vi "Get points_pretrigger_box.vi"(7 "level":dbl=3.0 format="%#_13g", 8 "error in (no error)":errorcluster, 9 "Sample Rate":dbl=1000000.0 format="%.3p", 10 "Voltage Read":tag="Dev1/ai1") -> (0 "error out":errorcluster, 3 "data":dbl[](array[numeric]) format="%0.2f")   [LabVIEW 2017]
uses:
  <vilib>/DAQmx/read.llb/DAQmx Read (Analog 1D DBL 1Chan NSamp).vi
  <vilib>/DAQmx/create/channels.llb/DAQmx Create Channel (AI-Voltage-Basic).vi
  <vilib>/DAQmx/configure/timing.llb/DAQmx Timing (Sample Clock).vi
  <vilib>/DAQmx/configure/trigger.llb/DAQmx Reference Trigger (Analog Edge).vi
  <vilib>/DAQmx/miscellaneous.llb/DAQmx Fill In Error Info.vi
panel:
  out "Waveform Graph":dbl[](graph)
  out "relative seconds 2":dbl format="%_19f"
  out "relative seconds":dbl format="%_19f"
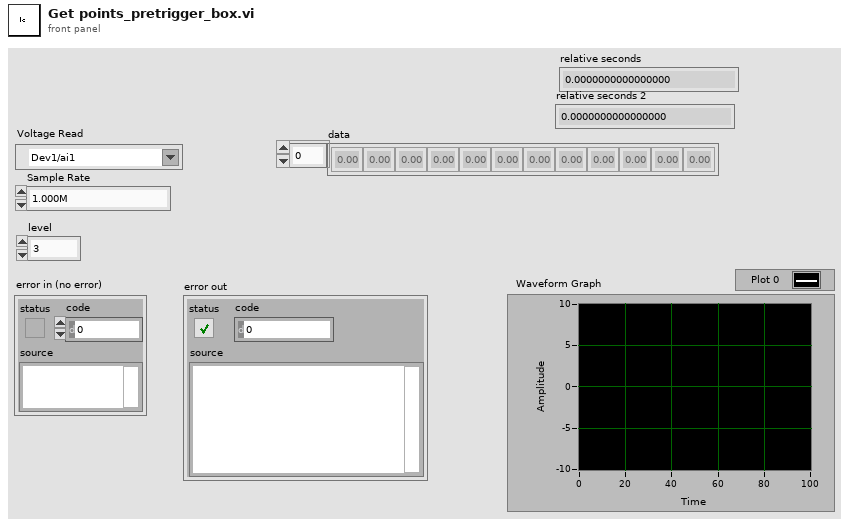
[diagram p1: front panel]
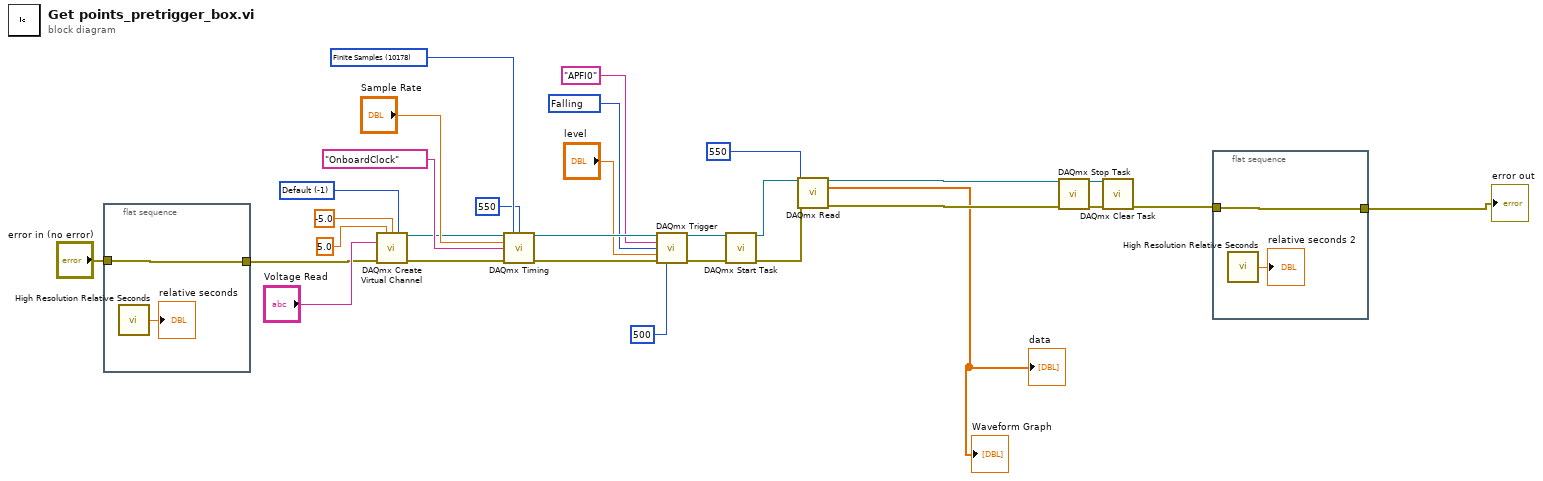
[diagram p0: block diagram]
diagram:
  w12 = 10171 items=["Rising"=10280, "Falling"=10171] ("slope")
  w24 = -1 items=["Default"=-1, "RSE"=10083, "NRSE"=10078, "Differential"=10106, "Pseudodifferential"=12529] ("input terminal configuration")
  w28 = 10178 items=["Finite Samples"=10178, "Continuous Samples"=10123, "Hardware Timed Single Point"=12522] ("sample mode")
  n1 = flat-sequence {
    tunnel: [w31] -> w6
    tunnel: "error in (no error)" -> [w31]
    frame #0 {
      n2 = call <vilib>:"High Resolution Relative Seconds.vi"() -> ("relative seconds"=→"relative seconds":dbl)
    }
  }
  n3 = call-poly <vilib>:"DAQmx Create Virtual Channel.vi"("maximum value"=5.0, "minimum value"=-5.0, "input terminal configuration"=w24, "physical channels"="Voltage Read", "error in"=w6) -> ("task out"=w23:refnum<k21>, "error out"=w22:errorcluster)  [unwired: 9 in]
  n4 = call-poly <vilib>:"DAQmx Timing.vi"("task/channels in"=w23, "sample mode"=w28, "samples per channel"=550, "rate"="Sample Rate", "source"=tag "OnboardClock", "error in"=w22) -> ("task out"=w15:refnum<k21>, "error out"=w21:errorcluster)  [unwired: 8 in]
  n5 = call-poly <vilib>:"DAQmx Trigger.vi"("task/channels in"=w15, "source"="APFI0", "slope"=w12, "level"="level", "error in"=w21, "pretrigger samples per channel"=u32 500) -> ("task out"=w20:refnum<k21>, "error out"=w19:errorcluster)  [unwired: 8 in]
  n6 = call <vilib>:"DAQmx Start Task.vi"("task/channels in"=w20, "error in"=w19) -> ("task out"=w18:refnum<k21>, "error out"=w9:errorcluster)  [unwired: 12 in]
  n7 = call-poly <vilib>:"DAQmx Read.vi"("task/channels in"=w18, "number of samples per channel"=550, "error in"=w9) -> ("task out"=w11:refnum<k21>, "data"=→"data" →"Waveform Graph":dbl[], "error out"=w10:errorcluster)  [unwired: 10 in]
  n8 = call <vilib>:"DAQmx Stop Task.vi"("task/channels in"=w11, "error in"=w10) -> ("task out"=w17:refnum<k21>, "error out"=w16:errorcluster)  [unwired: 12 in]
  n9 = call <vilib>:"DAQmx Clear Task.vi"("task in"=w17, "error in"=w16) -> ("error out"=w4:errorcluster)  [unwired: 13 in]
  n10 = flat-sequence {
    tunnel: [w33] -> w3
    tunnel: w4 -> [w33]
    frame #0 {
      n11 = call <vilib>:"High Resolution Relative Seconds.vi"() -> ("relative seconds"=→"relative seconds 2":dbl)
    }
  }
  "error out" <- w3
